vi "onIncomingMessagingError.vi"(8 "error in (no error)":errorcluster, 11 "ContextThisComponent in":refnum<class "ContextThisComponent.lvclass">) -> (0 "error out":errorcluster, 3 "ContextThisComponent out":refnum<class "ContextThisComponent.lvclass">)   [LabVIEW 2012, in "ContextThisComponent.lvclass"]
uses:
  ContextThisComponent.lvclass
  ContextThisComponent.lvclass/ContextThisComponent.ctl
  IStateFactory/IStateFactory.lvclass
  IModel/IModel.lvclass
  State/State.lvclass
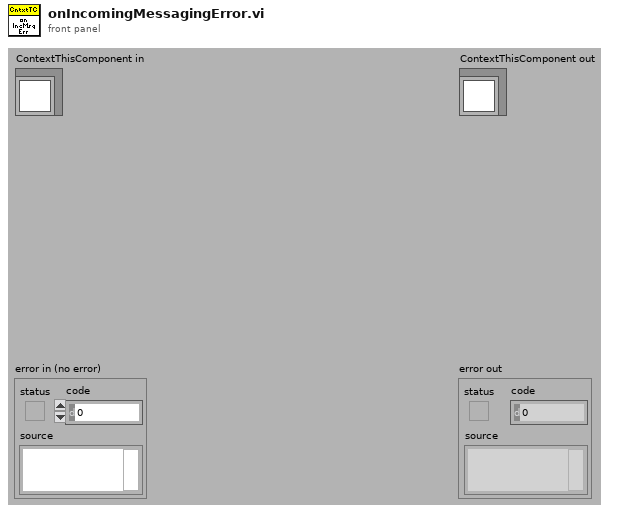
[diagram p1: front panel]
types:
  T1 = typedef "EXATypedefs.lvlib/StateValue.ctl" = enum16{"DisabledState", "EnabledState", "FaultState", "OffState", "StandbyState"}
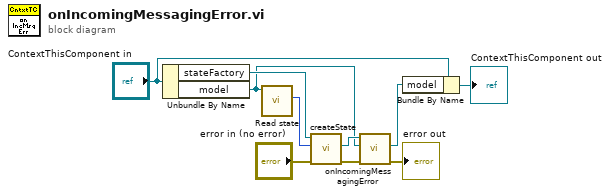
[diagram p0: block diagram]
diagram:
  n1 = Unbundle By Name("ContextThisComponent in") -> ("stateFactory"=w4:refnum<class "IStateFactory.lvclass">, "model"=w2:refnum<class "IModel.lvclass">)
  n2 = call-dynamic "Read state.vi"("IModel in"=w2) -> ("StateValue"=w1:T1)  [unwired: 9 in, 1 out]
  n3 = call-dynamic "createState.vi"("error in (no error)"="error in (no error)", "stateValue"=w1, "IStateFactory in"=w4) -> ("error out"=w3:errorcluster, "state"=w6:refnum<class "State.lvclass">)  [unwired: 6 in, 1 out]
  n4 = call-dynamic "onIncomingMessagingError.vi"("error in (no error)"=w3, "model in"=w2, "State in"=w6) -> ("error out"=→"error out":errorcluster, "model out"=w5:refnum<class "IModel.lvclass">)  [unwired: 6 in, 1 out]
  n5 = Bundle By Name(cluster="ContextThisComponent in", "model"=w5) -> (→"ContextThisComponent out":refnum<class "ContextThisComponent.lvclass">)
